vi "Synx2Power.vi"(8 "error in (no error)":errorcluster, 11 "RingdownPlugin in":refnum<class "RingdownPlugin.lvclass">) -> (0 "error out":errorcluster, 1 "Reactive Power":dbl[][](array[numeric]), 2 "Active Power":dbl[][](array[numeric]), 3 "RingdownPlugin out":refnum<class "RingdownPlugin.lvclass">)   [LabVIEW 2017, in "AppPlugins.lvlib" / "RingdownPlugin.lvclass"]
uses:
  RingdownPlugin.lvclass
  C:/dev/Work/PARTF/Modules/AppPlugins/AppPluginBaseClass/AppPluginsBase.lvclass
  AppPluginBaseClass/AppPluginsBase.lvclass/AppPluginsBase.ctl
  RingdownPlugin.lvclass/RingdownPlugin.ctl
  AppPluginBaseClass/Accessors/Read clEvtReportArray.vi
  Accessors/Read RingdownConfig.vi
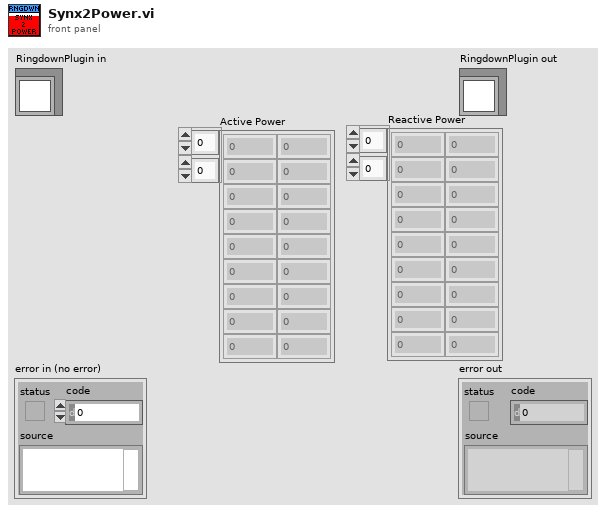
[diagram p1: front panel]
types:
  T1 = typedef "EventPlugins.lvlib/EventPluginBaseClass.lvclass/clEvtReportArray.ctl" = T2[]
  T2 = typedef "EventPlugins.lvlib/EventPluginBaseClass.lvclass/clEvtReport.ctl" = cluster{"Timestamp":dbl, "Synx":cdb[], "Freq":dbl, "ROCOF":dbl, "ID":i16}
  T3 = typedef "AppPlugins.lvlib/RingdownPlugin.lvclass/RingdownConfig.ctl" = cluster{"Config":cluster{"Addmod":i32, "Scalmod":i32, "Lpocon":i32, "Pircon":i32, "Dmodes":i32, "Lpmcon":u16, "Lpacon":u16, "Fbcon":u16, "Ordcon":i32, "Trimre":dbl, "Ftrimh":dbl, "Ftriml":dbl}, "Window":cluster{"StOffset":i32, "EndOffset":i32, "Length":i32}, "V index":i32, "I index":i32, "PosSeq":bool}
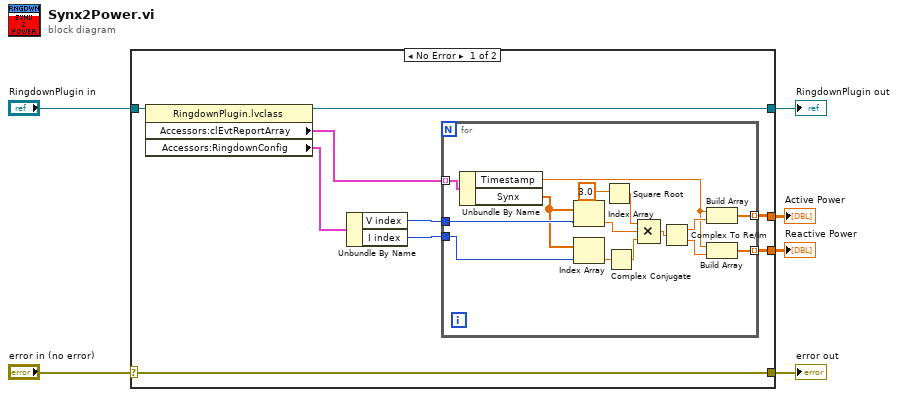
[diagram p0: block diagram]
diagram:
  n1 = case shown="No Error" "error in (no error)" {
    selector: "error in (no error)" -> [w14 w32]
    tunnel: [w14 w32] -> w5
    tunnel: [w13 w31] -> w3
    tunnel: "RingdownPlugin in" -> [w15 w31]
    tunnel: [w8 _] -> w2
    tunnel: [w7 _] -> w1
    frame No Error {
      n2 = property class="RingdownPlugin.lvclass"(reference=w15) -> (reference out=w13:refnum<class "RingdownPlugin.lvclass">, "Accessors:clEvtReportArray"=w9:T1, "Accessors:RingdownConfig"=w10:T3)  [unwired: 1 in, 1 out]
      n3 = Unbundle By Name(w10) -> ("V index"=w11:i32, "I index"=w12:i32)
      n4 = for {
        tunnel: w12 -> [w28]
        tunnel: w11 -> [w29]
        tunnel: w9 -> [w30] mode=indexing
        tunnel: [w19] -> w8 mode=indexing
        tunnel: [w18] -> w7 mode=indexing
        n5 = Unbundle By Name(w30) -> ("Timestamp"=w20:dbl, "Synx"=w27:cdb[])
        n6 = Index Array(array=w27, index=w29) -> (element=w24:cdb)
        n7 = Index Array(array=w27, index=w28) -> (element=w26:cdb)
        n8 = Square Root(x=3.0) -> (sqrt(x)=w17:dbl)
        n9 = Complex Conjugate(1:w26) -> (0:w25:cdb)
        n10 = Compound Arithmetic op=MULTIPLY(w17, w24, w25) -> (w23:cdb)
        n11 = Complex To Re/Im(x + iy=w23) -> (x=w21:dbl, y=w22:dbl)
        n12 = Build Array(w20, w21) -> (w19:dbl[])
        n13 = Build Array(w20, w22) -> (w18:dbl[])
      }
    }
    frame Error {
    }
  }
  "error out" <- w5
  "RingdownPlugin out" <- w3
  "Active Power" <- w2
  "Reactive Power" <- w1
